vi "Reactor Write Client.vi"() -> ()   [LabVIEW 2017]
uses:
  <vilib>/OPCUA/controls/Write Status.ctl
  <vilib>/OPCUA/controls/NodeId.ctl
  <vilib>/OPCUA/client/Multiple Write Double Array.vi
  <vilib>/OPCUA/client/Multiple Write Bool Array.vi
  <vilib>/OPCUA/client/Multiple Write String Array.vi
  <vilib>/OPCUA/NI OPC UA Client.lvlib
panel:
  in  "error in (no error)":errorcluster
  in  "Stop Reactor Digital Control":bool
  in  "Node Status":T1 items=["Good"=0, "Uncertain_InitialValue"=1083310080, "Uncertain_LastUsableValue"=1083179008, "Uncertain_SensorNotAccurate"=1083375616, "Uncertain_EngineeringUnitsExceeded"=1083441152, "Bad_NoCommunication"=2150694912, "Bad_NotReadable"=2151284736, "Bad_NotWritable"=2151350272, "Bad_OutOfRange"=2151415808, "Bad_WaitingForInitialData"=2150760448]
  in  "Time Stamp":timestamp
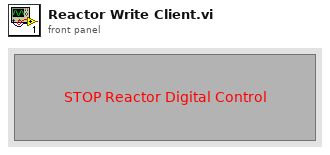
[diagram p1: front panel]
types:
  T1 = typedef "Write Status.ctl" = u32
  T2 = cluster{"message mode":enum16{"None", "Sign", "Sign and Encrypt"}, "security":enum16{"Basic256", "Basic128Rsa15"}}
  T3 = typedef "OPC UA Client Refnum.ctl" = refnum<k21>
  T4 = typedef "NodeId.ctl" = string
  T5 = cluster{"node ID":T4, "value":string[], "timestamp (current time)":timestamp, "node status":T1}
  T6 = cluster{"node ID":T4, "value":bool[], "timestamp (current time)":timestamp, "node status":T1}
  T7 = cluster{"node ID":T4, "value":dbl[], "timestamp (current time)":timestamp, "node status":T1}
  T8 = cluster{"node ID":T4, "value":dbl[], "timestamp (current time)":timestamp, "node status":T1}[]
  T9 = cluster{"node ID":T4, "value":bool[], "timestamp (current time)":timestamp, "node status":T1}[]
  T10 = cluster{"node ID":T4, "value":string[], "timestamp (current time)":timestamp, "node status":T1}[]
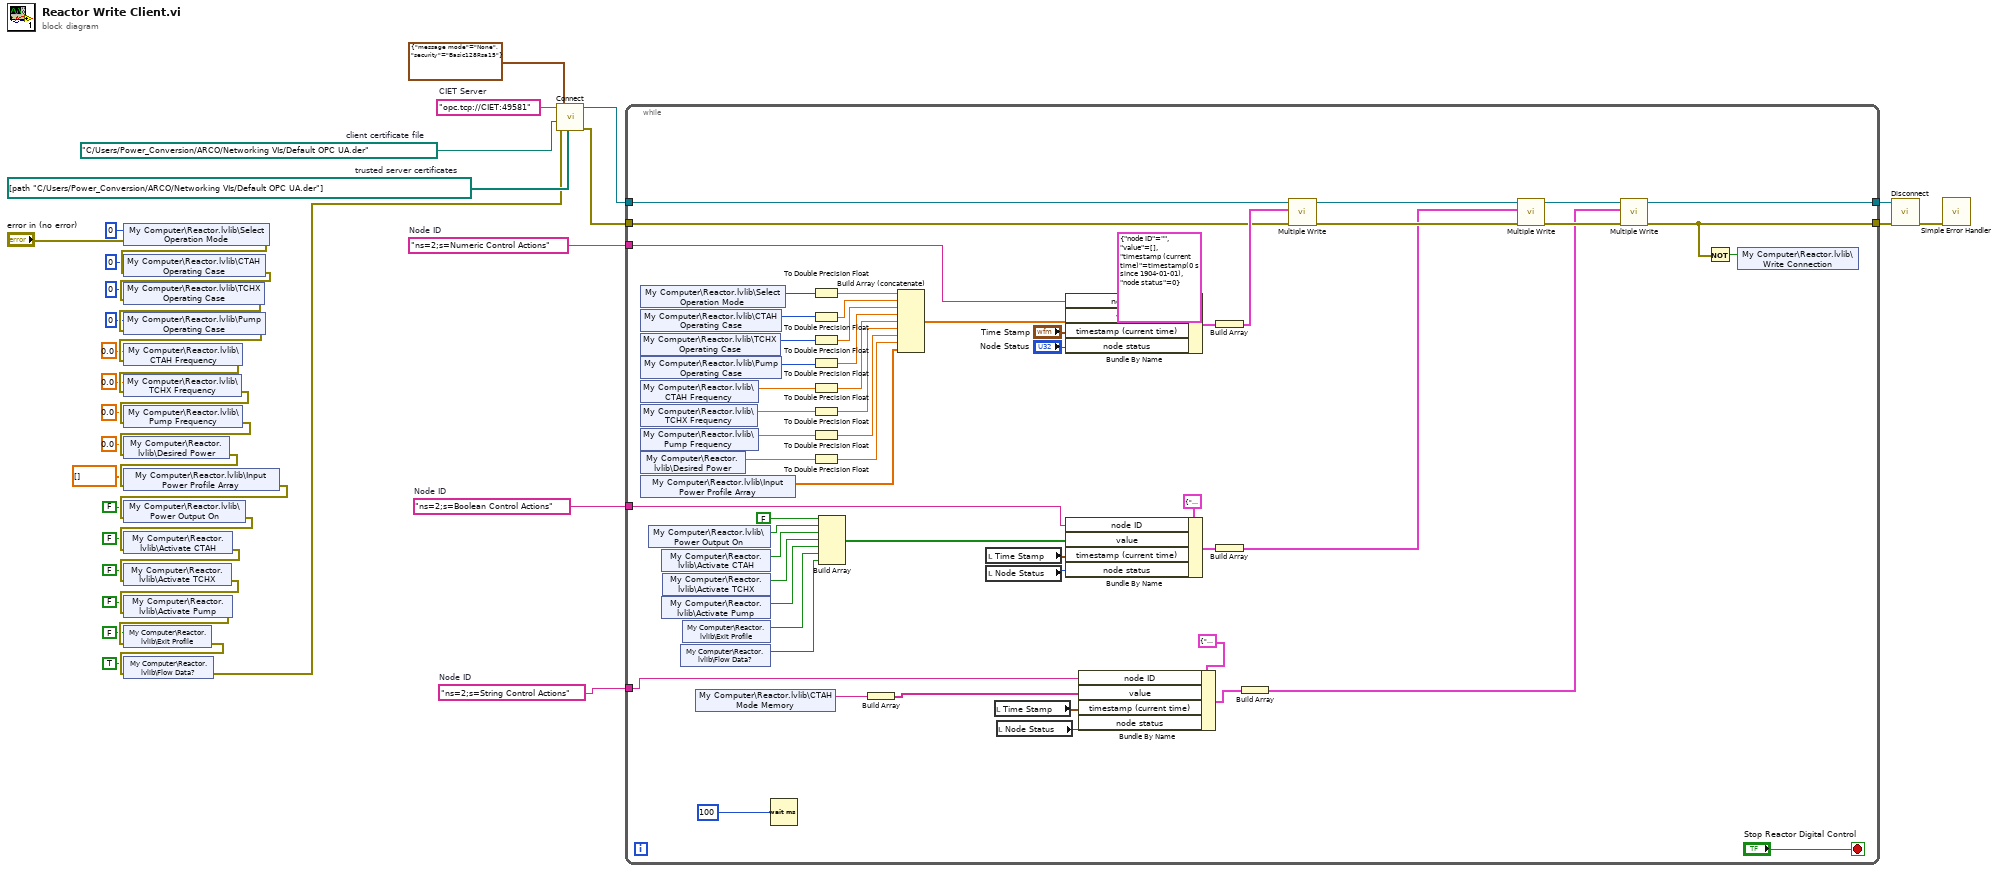
[diagram p0: block diagram]
diagram:
  w1 = "ns=2;s=String Control Actions"  # Node ID
  w36 = "ns=2;s=Boolean Control Actions"  # Node ID
  w37 = "ns=2;s=Numeric Control Actions"  # Node ID
  w40 = path[] [path "C:/Users/Power_Conversion/ARCO/Networking VIs/Default OPC UA.der"]  # trusted server certificates
  w41 = path "C:/Users/Power_Conversion/ARCO/Networking VIs/Default OPC UA.der"  # client certificate file
  w43 = "opc.tcp://CIET:49581"  # CIET Server
  n1 = shared-variable "My Computer\\Reactor.lvlib\\Select Operation Mode"(u16 0 ("Select Operation Mode"), error in="error in (no error)") -> (error out=w31:errorcluster)
  n2 = shared-variable "My Computer\\Reactor.lvlib\\CTAH Operating Case"(0 ("CTAH Operating Case"), error in=w31) -> (error out=w30:errorcluster)
  n3 = shared-variable "My Computer\\Reactor.lvlib\\TCHX Operating Case"(0 ("TCHX Operating Case"), error in=w30) -> (error out=w29:errorcluster)
  n4 = shared-variable "My Computer\\Reactor.lvlib\\Pump Operating Case"(0 ("Pump Operating Case"), error in=w29) -> (error out=w28:errorcluster)
  n5 = shared-variable "My Computer\\Reactor.lvlib\\CTAH Frequency"(sgl 0.0 ("CTAH Frequency"), error in=w28) -> (error out=w27:errorcluster)
  n6 = shared-variable "My Computer\\Reactor.lvlib\\TCHX Frequency"(sgl 0.0 ("TCHX Frequency"), error in=w27) -> (error out=w26:errorcluster)
  n7 = shared-variable "My Computer\\Reactor.lvlib\\Pump Frequency"(sgl 0.0 ("Pump Frequency"), error in=w26) -> (error out=w25:errorcluster)
  n8 = shared-variable "My Computer\\Reactor.lvlib\\Desired Power"(sgl 0.0 ("Desired Power"), error in=w25) -> (error out=w24:errorcluster)
  n9 = shared-variable "My Computer\\Reactor.lvlib\\Input Power Profile Array"(dbl[] [] ("Input Power Profile Array"), error in=w24) -> (error out=w23:errorcluster)
  n10 = shared-variable "My Computer\\Reactor.lvlib\\Power Output On"(FALSE ("Power Output On"), error in=w23) -> (error out=w22:errorcluster)
  n11 = shared-variable "My Computer\\Reactor.lvlib\\Activate CTAH"(FALSE ("Activate CTAH"), error in=w22) -> (error out=w21:errorcluster)
  n12 = shared-variable "My Computer\\Reactor.lvlib\\Activate TCHX"(FALSE ("Activate TCHX"), error in=w21) -> (error out=w20:errorcluster)
  n13 = shared-variable "My Computer\\Reactor.lvlib\\Activate Pump"(FALSE ("Activate Pump"), error in=w20) -> (error out=w19:errorcluster)
  n14 = shared-variable "My Computer\\Reactor.lvlib\\Exit Profile"(FALSE ("Exit Profile"), error in=w19) -> (error out=w18:errorcluster)
  n15 = shared-variable "My Computer\\Reactor.lvlib\\Flow Data?"(TRUE ("Flow Data?"), error in=w18) -> (error out=w17:errorcluster)
  n16 = call <vilib>:"Connect.vi"("trusted server certificates"=w40, "error in (no error)"=w17, "client certificate file"=w41, "security policy"=T2 {"message mode"=enum."None", "security"=enum."Basic128Rsa15"}, "server endpoint URL"=w43) -> ("error out"=w38:errorcluster, "OPC UA client refnum out"=w39:T3)  [unwired: 4 in, 1 out]
  n17 = while {
    tunnel: w39 -> [w81]
    tunnel: w38 -> [w79]
    tunnel: w37 -> [w69]
    tunnel: w36 -> [w68]
    tunnel: [w48] -> w35
    tunnel: [w46] -> w34
    tunnel: w1 -> [w51]
    stop <- "Stop Reactor Digital Control" stop-if-true
    n18 = shared-variable "My Computer\\Reactor.lvlib\\Select Operation Mode"() -> (w100:u16)  [unwired: 1 in, 1 out]
    n19 = shared-variable "My Computer\\Reactor.lvlib\\CTAH Operating Case"() -> (w97:i32)  [unwired: 1 in, 1 out]
    n20 = shared-variable "My Computer\\Reactor.lvlib\\TCHX Operating Case"() -> (w98:i32)  [unwired: 1 in, 1 out]
    n21 = shared-variable "My Computer\\Reactor.lvlib\\Pump Operating Case"() -> (w99:i32)  [unwired: 1 in, 1 out]
    n22 = shared-variable "My Computer\\Reactor.lvlib\\CTAH Frequency"() -> (w65:sgl)  [unwired: 1 in, 1 out]
    n23 = shared-variable "My Computer\\Reactor.lvlib\\TCHX Frequency"() -> (w64:sgl)  [unwired: 1 in, 1 out]
    n24 = shared-variable "My Computer\\Reactor.lvlib\\Pump Frequency"() -> (w63:sgl)  [unwired: 1 in, 1 out]
    n25 = shared-variable "My Computer\\Reactor.lvlib\\Desired Power"() -> (w62:sgl)  [unwired: 1 in, 1 out]
    n26 = shared-variable "My Computer\\Reactor.lvlib\\Input Power Profile Array"() -> (w57:dbl[])  [unwired: 1 in, 1 out]
    n27 = shared-variable "My Computer\\Reactor.lvlib\\Power Output On"() -> (w91:bool)  [unwired: 1 in, 1 out]
    n28 = shared-variable "My Computer\\Reactor.lvlib\\Activate CTAH"() -> (w90:bool)  [unwired: 1 in, 1 out]
    n29 = shared-variable "My Computer\\Reactor.lvlib\\Activate Pump"() -> (w88:bool)  [unwired: 1 in, 1 out]
    n30 = shared-variable "My Computer\\Reactor.lvlib\\Activate TCHX"() -> (w89:bool)  [unwired: 1 in, 1 out]
    n31 = shared-variable "My Computer\\Reactor.lvlib\\Flow Data?"() -> (w86:bool)  [unwired: 1 in, 1 out]
    n32 = shared-variable "My Computer\\Reactor.lvlib\\Exit Profile"() -> (w87:bool)  [unwired: 1 in, 1 out]
    n33 = shared-variable "My Computer\\Reactor.lvlib\\CTAH Mode Memory"() -> (w55:string)  [unwired: 1 in, 1 out]
    n34 = Wait (ms)(milliseconds to wait=u32 100) -> ()  [unwired: 1 out]
    n35 = To Double Precision Float(number=w100) -> (double precision float=w96:dbl)
    n36 = To Double Precision Float(number=w97) -> (double precision float=w95:dbl)
    n37 = To Double Precision Float(number=w98) -> (double precision float=w94:dbl)
    n38 = To Double Precision Float(number=w99) -> (double precision float=w93:dbl)
    n39 = To Double Precision Float(number=w65) -> (double precision float=w61:dbl)
    n40 = To Double Precision Float(number=w64) -> (double precision float=w60:dbl)
    n41 = To Double Precision Float(number=w63) -> (double precision float=w59:dbl)
    n42 = To Double Precision Float(number=w62) -> (double precision float=w58:dbl)
    n43 = Build Array(FALSE, w91, w90, w89, w88, w87, w86) -> (w74:bool[])
    n44 = Build Array(w55) -> (w50:string[])
    n45 = Build Array (concatenate)(w96, w95, w94, w93, w61, w60, w59, w58, w57) -> (w84:dbl[])
    n46 = local read "Time Stamp"() -> (w71:timestamp)
    n47 = local read "Node Status"() -> (w70:T1)
    n48 = local read "Time Stamp"() -> (w54:timestamp)
    n49 = local read "Node Status"() -> (w53:T1)
    n50 = Bundle By Name(cluster=T7 {"node ID"="", "value"=[], "timestamp (current time)"=timestamp(0 s since 1904-01-01), "node status"=0} ("request"), "node ID"=w69, "value"=w84, "timestamp (current time)"="Time Stamp", "node status"="Node Status") -> (w83:T7)
    n51 = Bundle By Name(cluster=T6 {"node ID"="", "value"=[], "timestamp (current time)"=timestamp(0 s since 1904-01-01), "node status"=0} ("request"), "node ID"=w68, "value"=w74, "timestamp (current time)"=w71, "node status"=w70) -> (w76:T6)
    n52 = Bundle By Name(cluster=T5 {"node ID"="", "value"=[], "timestamp (current time)"=timestamp(0 s since 1904-01-01), "node status"=0} ("request"), "node ID"=w51, "value"=w50, "timestamp (current time)"=w54, "node status"=w53) -> (w45:T5)
    n53 = Build Array(w83) -> (w82:T8)
    n54 = Build Array(w76) -> (w75:T9)
    n55 = Build Array(w45) -> (w44:T10)
    n56 = call-poly <vilib>:"Multiple Write.vi"("error in (no error)"=w79, "requests"=w82, "OPC UA client refnum in"=w81) -> ("error out"=w78:errorcluster, "OPC UA client refnum out"=w80:T3)  [unwired: 5 in, 2 out]
    n57 = call-poly <vilib>:"Multiple Write.vi"("error in (no error)"=w78, "requests"=w75, "OPC UA client refnum in"=w80) -> ("error out"=w47:errorcluster, "OPC UA client refnum out"=w49:T3)  [unwired: 5 in, 2 out]
    n58 = call-poly <vilib>:"Multiple Write.vi"("error in (no error)"=w47, "requests"=w44, "OPC UA client refnum in"=w49) -> ("error out"=w46:errorcluster, "OPC UA client refnum out"=w48:T3)  [unwired: 5 in, 2 out]
    n59 = Not(x=w46) -> (.not. x?=w56:bool)
    n60 = shared-variable "My Computer\\Reactor.lvlib\\Write Connection"(w56) -> ()  [unwired: 1 in, 1 out]
  }
  n61 = call <vilib>:"Disconnect.vi"("error in (no error)"=w34, "OPC UA client refnum in"=w35) -> ("error out"=w33:errorcluster)  [unwired: 9 in]
  n62 = call <vilib>:"Simple Error Handler.vi"("error in (no error)"=w33) -> ()  [unwired: 4 in, 5 out]
